vi "Create Client.vi"(7 "auto cleanup":bool=TRUE, 8 "error in":errorcluster, 10 "certificatePath":string, 11 "address":string) -> (0 "error out":errorcluster, 3 "gRPC ID Out":T1)   [LabVIEW 2021, in "Measurement Service Client V2.lvlib"]
uses:
  Measurement Service Client V2.lvlib
  <vilib>/gRPC/LabVIEW gRPC Library/Shared/grpcId.ctl
  <vilib>/gRPC/LabVIEW gRPC Library/grpc-lvsupport-release.lvlib
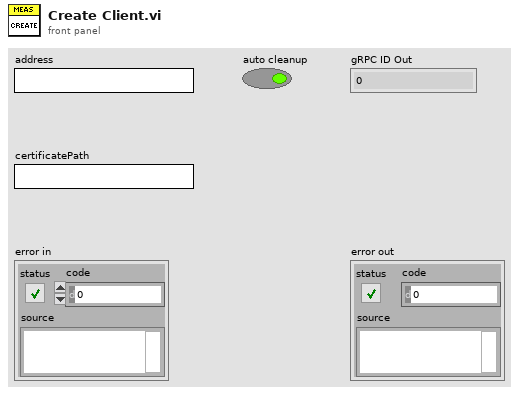
[diagram p1: front panel]
types:
  T1 = typedef "grpc-lvsupport-release.lvlib/grpcId.ctl" = u64
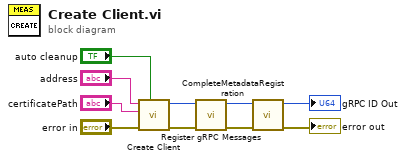
[diagram p0: block diagram]
diagram:
  n1 = call <vilib>:"Create Client.vi"("auto cleanup"="auto cleanup", "error in"="error in", "certificate path"="certificatePath", "address"="address") -> ("error out"=w6:errorcluster, "ClientID out"=w5:T1)  [unwired: 6 in]
  n2 = call "Register gRPC Messages.vi"("error in (no error)"=w6, "gRPC ID"=w5) -> ("error out"=w3:errorcluster, "gRPC ID Out"=w4:T1)  [unwired: 8 in]
  n3 = call <vilib>:"CompleteMetadataRegistration.vi"("error in"=w3, "gRPC ID in"=w4) -> ("error out"=→"error out":errorcluster, "gRPC ID Out"=→"gRPC ID Out":T1)  [unwired: 8 in]
